vi "destroy.vi"(8 "error in (no error)":errorcluster, 11 "Camera View in":refnum<class "Camera View.lvclass">) -> (0 "error out":errorcluster, 3 "Camera View out":refnum<class "Camera View.lvclass">)   [LabVIEW 2022 SP3, in "Camera View.lvclass"]
uses:
  Camera View.lvclass
  Camera View.lvclass/Camera View.ctl
  iView/base view/base view.lvclass
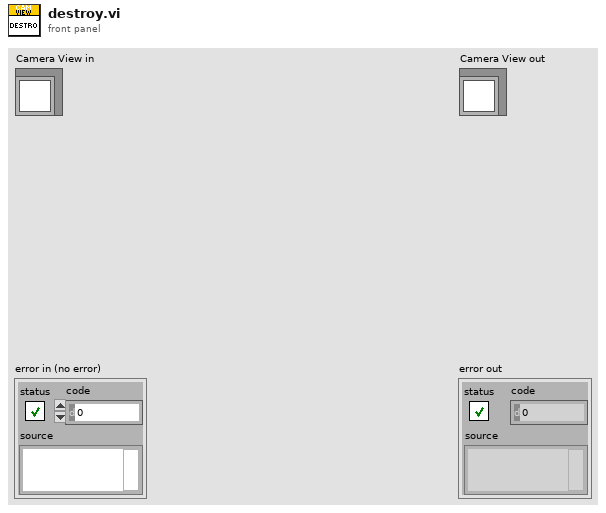
[diagram p1: front panel]
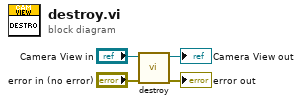
[diagram p0: block diagram]
diagram:
  n1 = call-parent "destroy.vi"("error in (no error)"="error in (no error)", "base view in"="Camera View in") -> ("error out"=→"error out":errorcluster, "base view out"=→"Camera View out":refnum<class "Camera View.lvclass">)  [unwired: 8 in]
